vi "CheckConnectivity.vi"(8 "error in (no error)":errorcluster, 11 "SiemensDigitalEnergyMeter in":refnum<class "SiemensDigitalEnergyMeter.lvclass">) -> (0 "error out":errorcluster, 2 "Are Any Connected?":bool, 3 "SiemensDigitalEnergyMeter out":refnum<class "SiemensDigitalEnergyMeter.lvclass">)   [LabVIEW 2018, in "SensorPlugins.lvlib" / "SiemensDigitalEnergyMeter.lvclass"]
doc: "This VI checks if communication has been sucessfully established between software and the instrument."
uses:
  SiemensDigitalEnergyMeter.lvclass
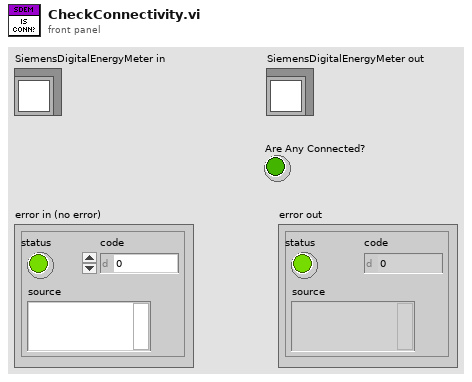
[diagram p1: front panel]
types:
  T1 = typedef "SensorPlugins.lvlib/SiemensDigitalEnergyMeter.lvclass/SiemensDigitalEnergyMeterControls.ctl" = cluster{"Measurement(s)":u16[], "Configuration Commands":string, "Use Measurement Commands Text Box?":bool, "Measurement Commands":string, "Connected?":bool, "Serial Number":string, "IP Address":string, "Port (502)":u16, "Unit ID":u8, "Serial Type":enum16{"RTU", "ASCII"}, "Using TCP?":bool, "VISA Resource Name":string}[]
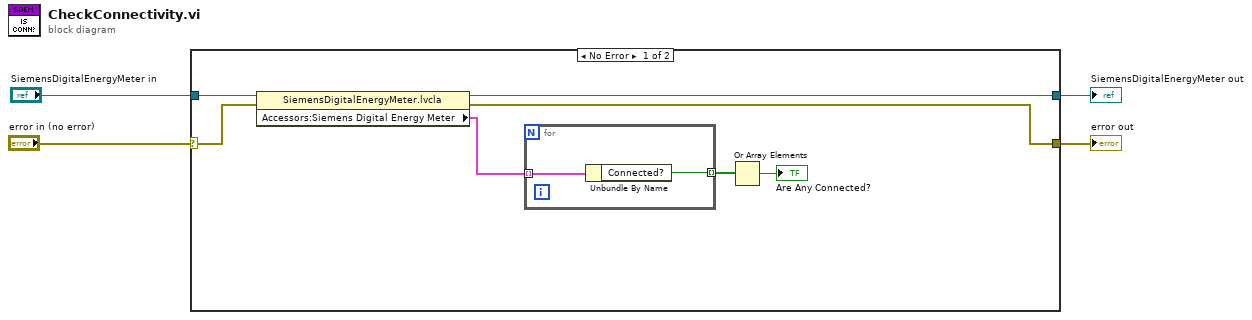
[diagram p0: block diagram]
diagram:
  n1 = case shown="No Error" "error in (no error)" {
    selector: "error in (no error)" -> [w9 w15]
    tunnel: "SiemensDigitalEnergyMeter in" -> [w11 w14]
    tunnel: [w8 w15] -> w2
    tunnel: [w10 w14] -> w1
    frame No Error {
      n2 = property class="SiemensDigitalEnergyMeter.lvcla"(reference=w11, error in=w9) -> (reference out=w10:refnum<class "SiemensDigitalEnergyMeter.lvclass">, error out=w8:errorcluster, "Accessors:Siemens Digital Energy Meter"=w7:T1)
      n3 = for {
        tunnel: w7 -> [w13] mode=indexing
        tunnel: [w12] -> w6 mode=indexing
        n4 = Unbundle By Name(w13) -> ("Connected?"=w12:bool)
      }
      n5 = Or Array Elements(Boolean array=w6) -> (logical OR=→"Are Any Connected?":bool)
    }
    frame Error {
    }
  }
  "error out" <- w2
  "SiemensDigitalEnergyMeter out" <- w1
